vi "Demo with Dynamic Data Types.vi"() -> ()   [LabVIEW 2016]
doc: "Demo showing dynamically changing data types and working with a tree.\n\nType Sensitive Popup \nCopyright © 2007, J. David Saunders\nAll rights reserved."
uses:
  <userlib>/TypeSens Popup/TSPopup.Popup Cluster.ctl
  <userlib>/TypeSens Popup/TSPopup.Data Type.ctl
  <userlib>/TypeSens Popup/TSPopup.Popup Call Parameters.ctl
panel:
  in  "Popups":T1 {"Boolean" items=["False", "True"]; "Ring" items=["Ring", "Elements", "to choose"]}
  in  "Test #":i32
  in  "Remove Param":bool
  in  "Show Popup (type only)":T2
  in  "Remove Test":bool
  in  "Add Test":bool
  in  "Add Param":bool
  in  "Parameter to Add to Test":T3=enum."Ring"
  in  "stop":bool
  in  "Tests":string(tree)
  # "Type Sensitive Popup \nCopyright © 2007, J. David Saunders\nAll rights reserved."
  # "Add parameters to existing tests, the popup automatically matches\nwhatever data type you specified.  Naturally one would have a\nconversion table between tag name and data type.  For convenience\nI just used the data type AS the tag name."
  # "Adding and removing parameters, as well as adding and removing tests\ndoesn't change how the Type Sensitive Popup behaves.  You just need\nto translate the tag you clicked on to the correct data type."
  # "Please ignore any errors in the adding and removing of Parameters/Tests."
  # "Type Sensitive\nPopup"
  # "Boolean Colors"
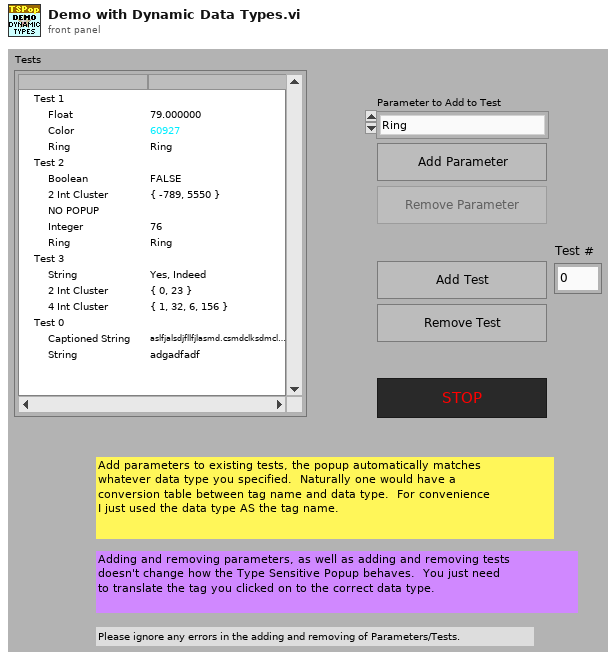
[diagram p1: front panel]
types:
  T1 = typedef "TSPopup.Popup Cluster.ctl" = cluster{"Unknown":bool, "Unknown 2":bool, "String":string, "Integer":i32, "Float":dbl, "Color":u32, "Boolean":u32, "Ring":u32, "Captioned String":cluster{"String":string, "OK":bool, "Cancel":bool}, "Captioned Integer":cluster{"First":i32, "OK":bool, "Cancel":bool}, "Boolean Colors":cluster{"False":cluster{"FG":u32, "BG":u32}, "True":cluster{"FG":u32, "BG":u32}, "T  to  F":cluster{"FG":u32, "BG":u32}, "F  to  T":cluster{"FG":u32, "BG":u32}, "OK":bool, "Cancel":bool}, "2-Int Cluster":cluster{"First":i32, "Second":i32, "OK":bool, "Cancel":bool}, "4-Int Cluster":cluster{"First":i32, "Second":i32, "Third":i32, "Fourth":i32, "OK":bool, "Cancel":bool}}
  T2 = typedef "TSPopup.Popup Call Parameters.ctl" = cluster{"Prop Type":T3, "Initial Value":variant, "Caption Strings":string[], "Ring Strings":string[], "Cell Rect":cluster{"left":i16, "top":i16, "right":i16, "bottom":i16}, "Mouse Coords":cluster{"x":i16, "y":i16}, "Call Data":variant}
  T3 = typedef "TSPopup.Data Type.ctl" = enum16{"Unkown", "NO POPUP", "String", "Integer", "Float", "Color", "Boolean", "Ring", "Captioned String", "Captioned Integer", "Button Color", "2 Int Cluster", "4 Int Cluster"}
  T4 = typedef "LVPoint32TypeDef.ctl" = cluster{"Horizontal":i32, "Vertical":i32}
  T5 = typedef "TSPopup.Grid.Cell Info.ctl" = cluster{"Tag":string, "Row":i32, "Column":i32, "In Symbol?":bool, "In Data?":bool, "Cell String":string, "Ctl Refnum":refnum<vi>, "Prop Type":T3, "Ring Strings":string[]}
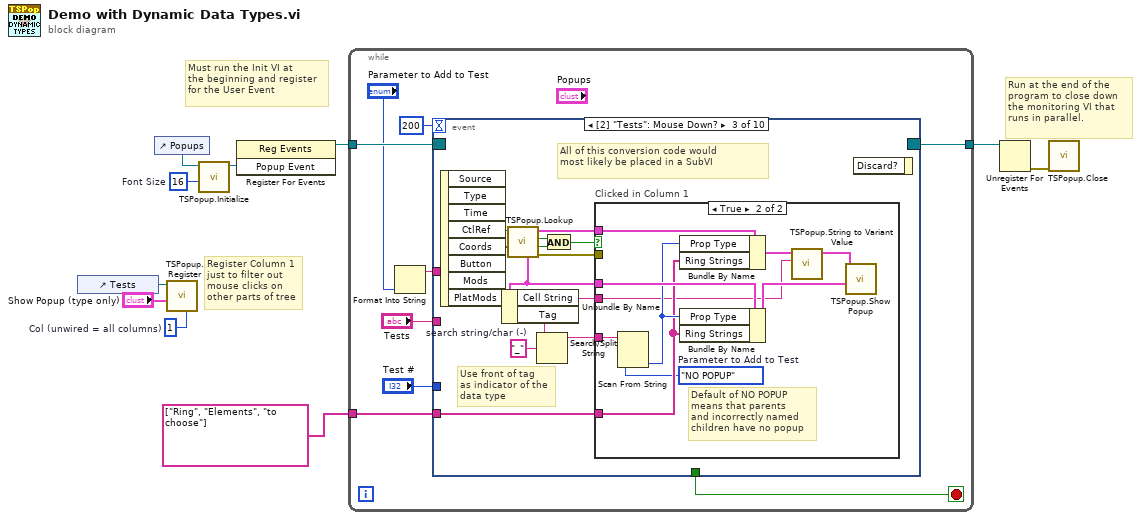
[diagram p0: block diagram]
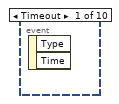
[diagram p2: hidden frame]
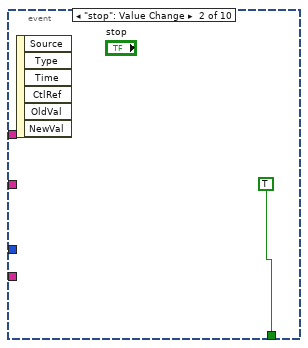
[diagram p3: hidden frame]
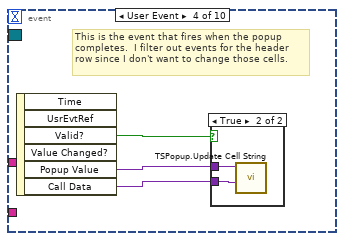
[diagram p5: hidden frame]
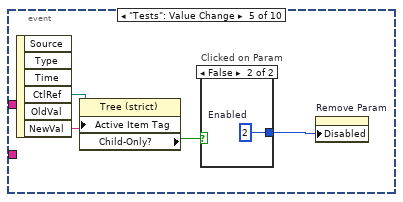
[diagram p7: hidden frame]
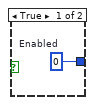
[diagram p8: hidden frame]
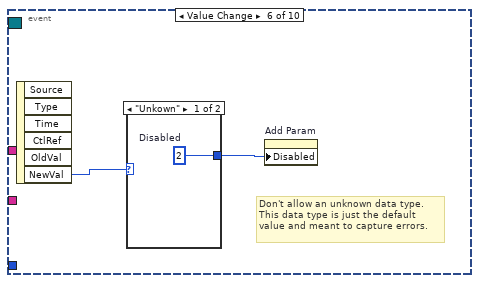
[diagram p9: hidden frame]
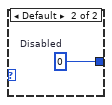
[diagram p10: hidden frame]
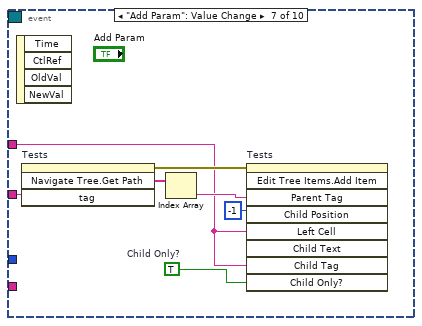
[diagram p11: hidden frame]
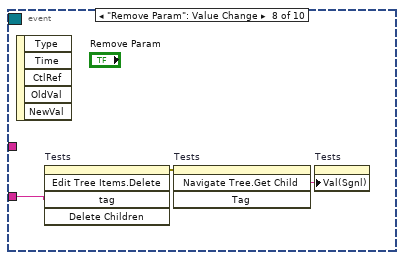
[diagram p12: hidden frame]
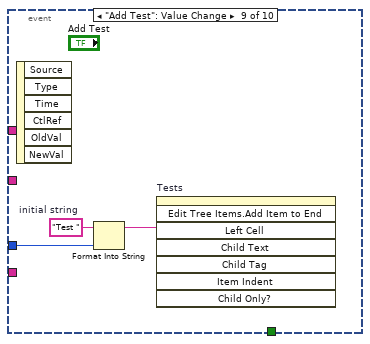
[diagram p13: hidden frame]
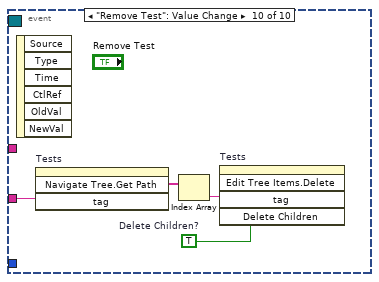
[diagram p14: hidden frame]
diagram:
  w3 = 1  # Col (unwired = all columns)
  w9 = u32 16  # Font Size
  # "Register Column 1\njust to filter out\nmouse clicks on\nother parts of tree"
  # "Run at the end of the\nprogram to close down\nthe monitoring VI that\nruns in parallel."
  # "Must run the Init VI at\nthe beginning and register\nfor the User Event"
  n1 = control-ref of="Tests"() -> (w4:refnum<vi>)
  n2 = control-ref of="Popups"() -> (w10:refnum<vi>)
  n3 = call <userlib>:"TSPopup.Register.vi"("Col (unwired = all columns)"=w3, "Parameters"="Show Popup (type only)", "Ctl Refnum"=w4) -> ()  [unwired: 7 in, 2 out]
  n4 = call <userlib>:"TSPopup.Initialize.vi"("Font Size"=w9, "Popup Cluster Ref"=w10) -> ("Popup Event"=w8:refnum<user-event>)  [unwired: 8 in, 1 out]
  n5 = register-events(w8) -> (reference out=w7:refnum<event-registration>)  [unwired: 2 in, 1 out]
  n6 = while {
    tunnel: w7 -> [w19]
    tunnel: [w18] -> w6
    tunnel: string[] ["Ring", "Elements", "to choose"] -> [w11]
    stop <- w17 stop-if-true
    n7 = Format Into String("Parameter to Add to Test") -> (resulting string=w14:string)  [unwired: 3 in, 1 out]
    n8 = event shown="[2] \"Tests\": Mouse Down?" {
      selector: w19 -> [_ _ _ _ _ _ _ _ _ _]
      dyn-events: [_ _ _ _ _ _ _ _ _ _] -> w18
      timeout: 200 -> [_ _ _ _ _ _ _ _ _ _]
      tunnel: [_ TRUE _ _ _ _ _ _ _ _] -> w17
      tunnel: "Tests" -> [_ _ _ _ _ _ w65 w68 _ w75]
      tunnel: w14 -> [_ _ _ _ _ _ w60 _ _ _]
      tunnel: "Test #" -> [_ _ _ _ _ _ _ _ w71 _]
      tunnel: w11 -> [_ _ w22 _ _ _ _ _ _ _]
      event Timeout {
        n9 = event-data() -> ()  [unwired: 1 in, 2 out]
      }
      event "stop": Value Change {
        n10 = event-data() -> ()  [unwired: 1 in, 6 out]
      }
      event "Tests": Mouse Down? {
        w24 = "_"  # search string/char (-)
        # "All of this conversion code would\nmost likely be placed in a SubVI"
        # "Use front of tag\nas indicator of the\ndata type"
        n11 = event-data() -> ("CtlRef"=w33:refnum<vi>, "Coords"=w32:T4)  [unwired: 1 in, 6 out]
        n12 = call <userlib>:"TSPopup.Lookup.vi"("Point"=w32, "Ctl Refnum"=w33) -> ("error out"=w27:errorcluster, "In Bounds?"=w30:bool, "Found"=w31:bool, "Popup Parameters"=w28:T2, "Cell Info (Call data)"=w26:T5)  [unwired: 5 in]
        n13 = Unbundle By Name(w26) -> ("Cell String"=w21:string, "Tag"=w25:string)
        n14 = Search/Split String(string=w25, search string/char (-)=w24) -> (substring before match=w23:string)  [unwired: 1 in, 2 out]
        n15 = And(x=w31, y=w30) -> (x .and. y?=w29:bool)
        n16 = case "Clicked in Column 1" shown="True" w29 {
          tunnel: w28 -> [_ w43]
          tunnel: w26 -> [_ w41]
          tunnel: w27 -> [_ _]
          tunnel: w23 -> [_ w42]
          tunnel: w22 -> [_ w38]
          tunnel: w21 -> [_ w35]
          frame False {
          }
          frame True {
            w37 = TSPopup.Data_Type."NO POPUP"  # Parameter to Add to Test
            # "Default of NO POPUP\nmeans that parents\nand incorrectly named\nchildren have no popup"
            n17 = Scan From String(input string=w42, default 1=w37) -> (output 1=w39:T3)  [unwired: 3 in, 3 out]
            n18 = Bundle By Name(cluster=w43, "Prop Type"=w39, "Ring Strings"=w38) -> (w36:T2)
            n19 = Bundle By Name(cluster=w41, "Prop Type"=w39, "Ring Strings"=w38) -> (w40:T5)
            n20 = call <userlib>:"TSPopup.String to Variant Value.vi"("Cell String"=w35, "Popup Parameters"=w36) -> ("Popup Parameters out"=w34:T2)  [unwired: 7 in, 2 out]
            n21 = call <userlib>:"TSPopup.Show Popup.vi"("Call Data (ignore if empty)"=w40, "Popup Parameters"=w34) -> ()  [unwired: 9 in, 1 out]
          }
        }
        n22 = event-data() -> ()  [unwired: 2 in, 1 out]
      }
      event User Event {
        # "This is the event that fires when the popup\ncompletes.  I filter out events for the header\nrow since I don't want to change those cells."
        n23 = event-data() -> ("Valid?"=w46:bool, "Popup Value"=w45:variant, "Call Data"=w44:variant)  [unwired: 1 in, 3 out]
        n24 = case shown="True" w46 {
          tunnel: w45 -> [_ w47]
          tunnel: w44 -> [_ w48]
          frame False {
          }
          frame True {
            n25 = call <userlib>:"TSPopup.Update Cell String.vi"("Call Data (must be Cell Info cluster)"=w48, "Popup Value"=w47) -> ()  [unwired: 9 in, 1 out]
          }
        }
      }
      event "Tests": Value Change {
        n26 = event-data() -> ("CtlRef"=w52:refnum<vi>, "NewVal"=w51:string)  [unwired: 1 in, 4 out]
        n27 = property class="Tree (strict)"(reference=w52, "Active Item Tag"=w51) -> ("Child-Only?"=w50:bool)  [unwired: 1 in, 2 out]
        n28 = case "Clicked on Param" shown="False" w50 {
          tunnel: [w53 w54] -> w49
          frame True {
            w53 = u8 0  # Enabled
          }
          frame False {
            w54 = u8 2  # Enabled
          }
        }
        n29 = property on="Remove Param" class="Bool"("Disabled"=w49) -> ()  [unwired: 2 in, 2 out]
      }
      event Value Change {
        # "Don't allow an unknown data type.\nThis data type is just the default\nvalue and meant to capture errors."
        n30 = event-data() -> ("NewVal"=w56:T3)  [unwired: 1 in, 5 out]
        n31 = case shown="\"Unkown\"" w56 {
          tunnel: [w57 w58] -> w55
          frame "Unkown" {
            w57 = u8 2  # Disabled
          }
          frame Default {
            w58 = u8 0  # Disabled
          }
        }
        n32 = property on="Add Param" class="Bool"("Disabled"=w55) -> ()  [unwired: 2 in, 2 out]
      }
      event "Add Param": Value Change {
        w59 = TRUE  # Child Only?
        n33 = event-data() -> ()  [unwired: 1 in, 4 out]
        n34 = invoke on="Tests" class="Tree (strict)" method="Navigate Tree.Get Path"("tag"=w65) -> (error out=w63:errorcluster, "Navigate Tree:Get Path"=w64:string[])  [unwired: 3 in, 2 out]
        n35 = Index Array(array=w64) -> (element=w62:string)  [unwired: 1 in]
        n36 = invoke on="Tests" class="Tree (strict)" method="Edit Tree Items.Add Item"(error in=w63, "Parent Tag"=w62, "Child Position"=-1, "Left Cell"=w60, "Child Tag"=w60, "Child Only?"=w59) -> ()  [unwired: 3 in, 9 out]
      }
      event "Remove Param": Value Change {
        n37 = event-data() -> ()  [unwired: 1 in, 5 out]
        n38 = invoke on="Tests" class="Tree (strict)" method="Edit Tree Items.Delete"("tag"=w68) -> (error out=w67:errorcluster)  [unwired: 4 in, 4 out]
        n39 = invoke on="Tests" class="Tree (strict)" method="Navigate Tree.Get Child"(error in=w67) -> ("Navigate Tree:Get Child"=w66:string)  [unwired: 3 in, 3 out]
        n40 = property on="Tests" class="Tree (strict)"("Val(Sgnl)"=w66) -> ()  [unwired: 2 in, 2 out]
      }
      event "Add Test": Value Change {
        w70 = "Test "  # initial string
        n41 = event-data() -> ()  [unwired: 1 in, 6 out]
        n42 = Format Into String(initial string=w70, w71) -> (resulting string=w69:string)  [unwired: 2 in, 1 out]
        n43 = invoke on="Tests" class="Tree (strict)" method="Edit Tree Items.Add Item to End"("Left Cell"=w69) -> ()  [unwired: 7 in, 8 out]
      }
      event "Remove Test": Value Change {
        w72 = TRUE  # Delete Children?
        n44 = event-data() -> ()  [unwired: 1 in, 6 out]
        n45 = invoke on="Tests" class="Tree (strict)" method="Navigate Tree.Get Path"("tag"=w75) -> ("Navigate Tree:Get Path"=w74:string[])  [unwired: 3 in, 3 out]
        n46 = Index Array(array=w74) -> (element=w73:string)  [unwired: 1 in]
        n47 = invoke on="Tests" class="Tree (strict)" method="Edit Tree Items.Delete"("tag"=w73, "Delete Children"=w72) -> ()  [unwired: 3 in, 5 out]
      }
    }
  }
  n48 = Unregister For Events(event registration refnum=w6) -> (error out=w5:errorcluster)  [unwired: 1 in]
  n49 = call <userlib>:"TSPopup.Close.vi"("error in (no error)"=w5) -> ()  [unwired: 10 in, 1 out]
